vi "GetRxPendingMsg.vi"(8 "error in (no error)":errorcluster, 11 "Konvolucio MCAN120803 Adapter Class in":refnum<class "Konvolucio MCAN120803 Adapter Class.lvclass">) -> (0 "error out":errorcluster, 2 "Value":i32, 3 "Konvolucio MCAN120803 Adapter Class out":refnum<class "Konvolucio MCAN120803 Adapter Class.lvclass">)   [LabVIEW 2011, in "Konvolucio MCAN120803 Adapter Class.lvclass"]
uses:
  Konvolucio MCAN120803 Adapter Class.lvclass
  Generic CAN Adapter/GenericCanAdapterClass.lvclass
  Konvolucio MCAN120803 Adapter Class.lvclass/Konvolucio MCAN120803 Adapter Class.ctl
  <instrlib>/Konvolucio MCAN120803/Konvolucio MCAN120803.lvlib
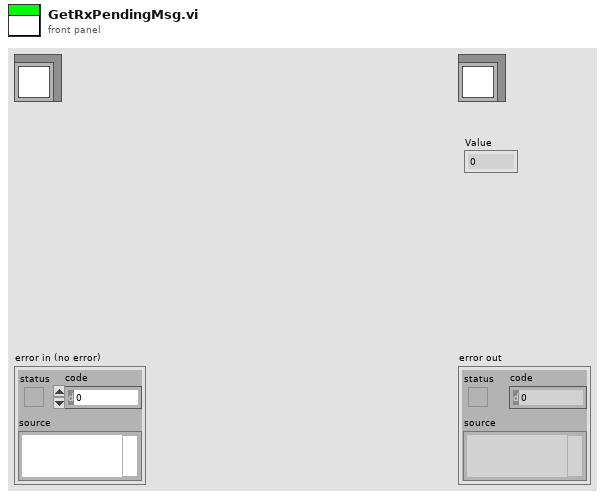
[diagram p1: front panel]
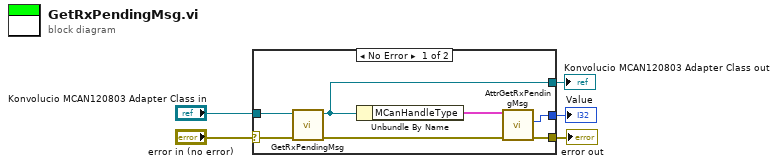
[diagram p0: block diagram]
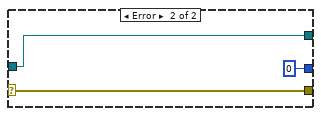
[diagram p2: hidden frame]
diagram:
  n1 = case shown="No Error" "error in (no error)" {
    selector: "error in (no error)" -> [w6 w15]
    tunnel: "Konvolucio MCAN120803 Adapter Class in" -> [w12 w14]
    tunnel: [w11 w14] -> w4
    tunnel: [w8 w15] -> w3
    tunnel: [w7 0 ("Value")] -> w2
    frame No Error {
      n2 = call-parent "GetRxPendingMsg.vi"("error in (no error)"=w6, "GenericCanAdapterClass in"=w12) -> ("error out"=w10:errorcluster, "GenericCanAdapterClass out"=w11:refnum<class "Konvolucio MCAN120803 Adapter Class.lvclass">)  [unwired: 7 in, 1 out]
      n3 = Unbundle By Name(w11) -> ("MCanHandleType"=w9:cluster{"MCanAdapter":refnum<k24>})
      n4 = call <instrlib>:"AttrGetRxPendingMsg.vi"("error in"=w10, "CanHandleIn"=w9) -> ("error out"=w8:errorcluster, "Value"=w7:i32)  [unwired: 7 in, 1 out]
    }
    frame Error {
    }
  }
  "error out" <- w3
  "Konvolucio MCAN120803 Adapter Class out" <- w4
  "Value" <- w2
